vi "FTW-ProjectItemManager-Destroy.vi"(0 "Project Item Manager":refnum<class "FTW-ProjectItemManager.lvclass">, 11 "error in":errorcluster) -> (15 "error out":errorcluster)   [LabVIEW 2012, in "FTW-ProjectItemManager.lvclass"]
uses:
  FTW-ProjectItemManager.lvclass
  FTW-ProjectItemManager.lvclass/FTW-ProjectItemManager.ctl
  Core/Messaging/Messenger.Actor/FTW-Messenger-Actor.lvclass
panel:
  # "Inputs"
  # "Outputs"
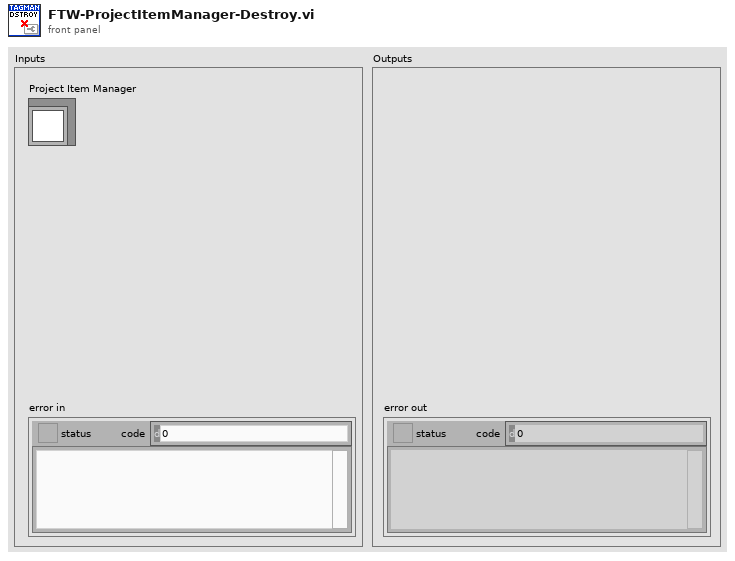
[diagram p1: front panel]
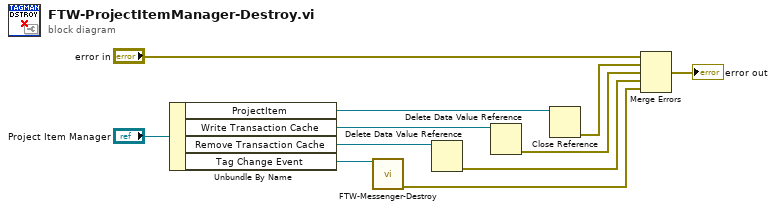
[diagram p0: block diagram]
diagram:
  n1 = Unbundle By Name("Project Item Manager") -> ("ProjectItem"=w6:refnum<vi>, "Write Transaction Cache"=w8:refnum<data-value>, "Remove Transaction Cache"=w2:refnum<data-value>, "Tag Change Event"=w4:refnum<class "FTW-Messenger-Actor.lvclass">)
  n2 = call-dynamic "FTW-Messenger-Destroy.vi"("Messenger"=w4) -> ("error out"=w3:errorcluster)  [unwired: 14 in]
  n3 = Delete Data Value Reference(data value reference=w2) -> (error out=w1:errorcluster)  [unwired: 1 in, 1 out]
  n4 = Delete Data Value Reference(data value reference=w8) -> (error out=w7:errorcluster)  [unwired: 1 in, 1 out]
  n5 = Close Reference(reference=w6) -> (error out=w5:errorcluster)  [unwired: 1 in]
  n6 = Merge Errors("error in", w5, w7, w1, w3) -> (→"error out":errorcluster)
